vi "ReverseByteExample.vi"(3 "Numeric":u8) -> (1 "Numeric 2":u8)   [LabVIEW 2026]
panel:
  out "Boolean array 2":bool[](array[boolean])
  out "Boolean array":bool[](array[boolean])
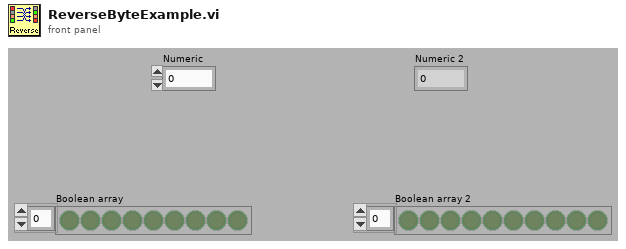
[diagram p1: front panel]
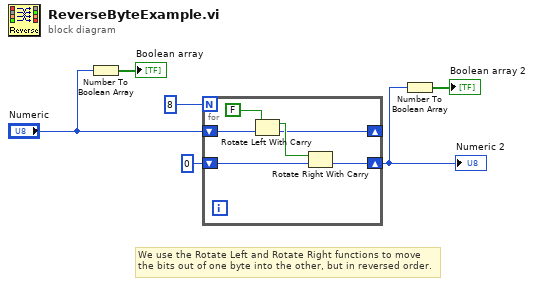
[diagram p0: block diagram]
diagram:
  # "We use the Rotate Left and Rotate Right functions to move the bits out of one byte into the other, but in reversed order."
  n1 = Number To Boolean Array(number="Numeric") -> (Boolean array=→"Boolean array":bool[])
  n2 = for {
    N: 8 -> [_]
    shift-right: [w8] -> _
    shift-left: "Numeric" -> [w12]
    shift-right: [w11] -> w2
    shift-left: u8 0 -> [w9]
    n3 = Rotate Left With Carry(2:w12, 3:FALSE ("carry")) -> (0:w8:u8, 1:w10:bool)
    n4 = Rotate Right With Carry(2:w9, 3:w10) -> (0:w11:u8)  [unwired: 1 out]
  }
  "Numeric 2" <- w2
  n5 = Number To Boolean Array(number=w2) -> (Boolean array=→"Boolean array 2":bool[])
